vi "Test gRPC cRIO XNET Read DBC Signals.vi"(11 "Test Case In":refnum<class "Test Communicator gRPC.lvclass">) -> (0 "error out":errorcluster, 3 "Test Case Out":refnum<class "Test Communicator gRPC.lvclass">)   [LabVIEW 2025, in "Test Communicator gRPC.lvclass"]
uses:
  Test Communicator gRPC.lvclass
  Test Communicator gRPC.lvclass/Test Communicator gRPC.ctl
  Source/Configure Strategies/gRPC XNET Read Raw CAN Frame Strategy/gRPC XNET Read Raw CAN Frame Strategy.lvclass
  D:/git/HAL/Source/Interfaces/IConfigure/IConfigure.lvclass
  D:/git/HAL/Source/Interfaces/IClose/IClose.lvclass
  D:/git/HAL/Source/Interfaces/IInitialize/IInitialize.lvclass
  D:/git/HAL/HAL-Devices/Source/Configure Strategies/gRPC XNET Read Raw CAN Frame Strategy/gRPC XNET Read Raw CAN Frame Strategy.lvclass
  D:/git/HAL/Source/Interfaces/ICommunicate/ICommunicate.lvclass
  D:/git/HAL/Source/Interfaces/IRunnable/IRunnable.lvclass
  C:/Program Files/National Instruments/LabVIEW 2025/vi.lib/Astemes/LUnit/Test Case.lvclass
  C:/Program Files/National Instruments/LabVIEW 2025/vi.lib/Astemes/LUnit/LUnit Runnable.lvclass
  D:/git/HAL/HAL-Devices/Tests/New folder/Test Communicator gRPC.lvclass
  <vilib>/Astemes/LUnit/Test Case.lvclass
  Source/DBC Communicator/DBC Communicator.lvclass
panel:
  out "Time Stamp":timestamp format="%<%x %.3X>T"
  out "Temp":dbl
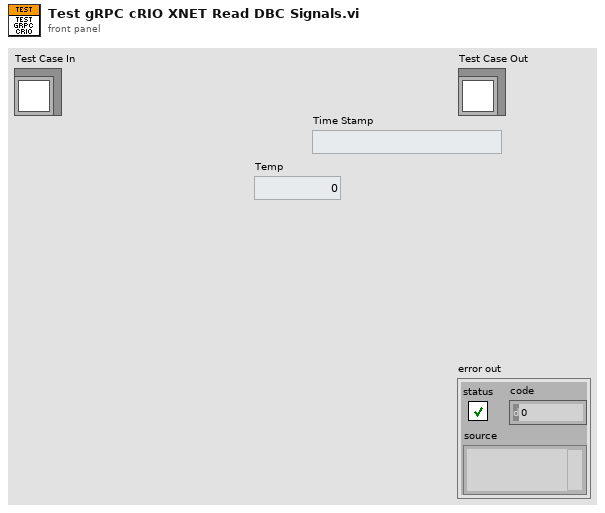
[diagram p1: front panel]
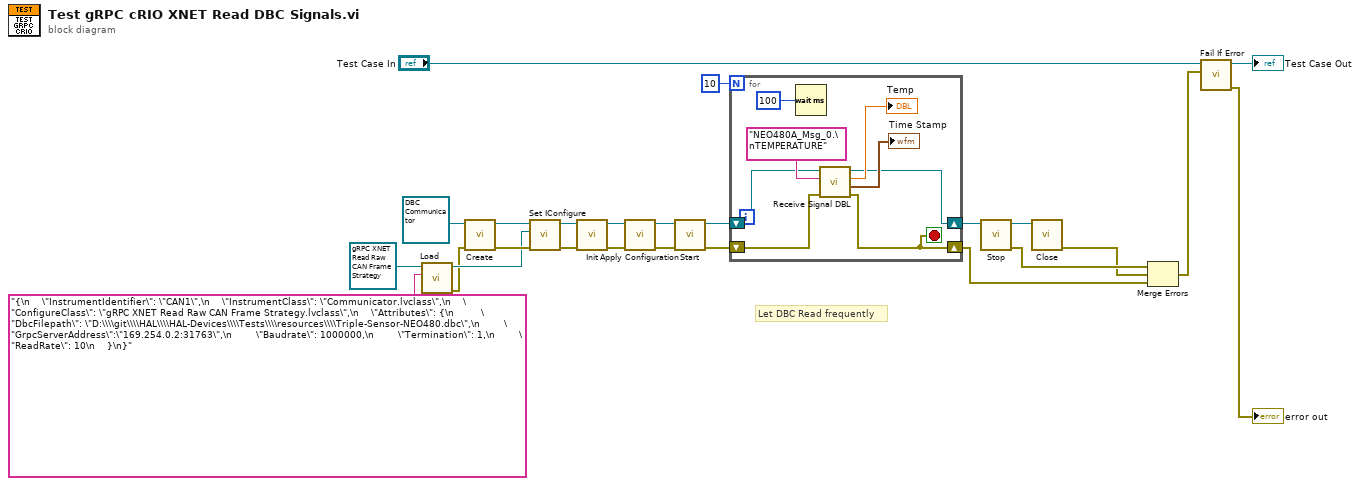
[diagram p0: block diagram]
diagram:
  # "Let DBC Read frequently"
  n1 = call-dynamic "Load.vi"("Source"="{\n    \"InstrumentIdentifier\": \"CAN1\",\n    \"InstrumentClass\": \"Communicator.lvclass\",\n    \"ConfigureClass\": \"gRPC XNET Read Raw CAN Frame Strategy.lvclass\",\n    \"Attributes\": {\n         \"DbcFilepath\": \"D:\\\\git\\\\HAL\\\\HAL-Devices\\\\Tests\\\\resources\\\\Triple-Sensor-NEO480.dbc\",\n        \"GrpcServerAddress\":\"169.254.0.2:31763\",\n        \"Baudrate\": 1000000,\n        \"Termination\": 1,\n        \"ReadRate\": 10\n    }\n}", "gRPC XNET Read Raw CAN Frame Strategy in"=refnum<class "gRPC XNET Read Raw CAN Frame Strategy.lvclass"> refnum ("IConfigure")) -> ("error out"=w8:errorcluster, "gRPC XNET Read Raw CAN Frame Strategy out"=w21:refnum<class "gRPC XNET Read Raw CAN Frame Strategy.lvclass">)  [unwired: 8 in]
  n2 = call-dynamic "Create.vi"("Error In"=w8, "reference in"=refnum<class "DBC Communicator.lvclass"> refnum ("Communicator in")) -> ("Error Out"=w22:errorcluster, "reference out"=w14:refnum<class "DBC Communicator.lvclass">)  [unwired: 8 in]
  n3 = call-dynamic "Set IConfigure.vi"("Error In"=w22, "IConfigure"=w21, "Communicator in"=w14) -> ("Error Out"=w19:errorcluster, "Communicator out"=w1:refnum<class "DBC Communicator.lvclass">)  [unwired: 7 in]
  n4 = call-dynamic "Init.vi"("Error In"=w19, "Communicator in"=w1) -> ("Error Out"=w18:errorcluster, "Communicator out"=w17:refnum<class "DBC Communicator.lvclass">)  [unwired: 8 in]
  n5 = call-dynamic "Apply Configuration.vi"("Error In"=w18, "reference in"=w17) -> ("Error Out"=w12:errorcluster, "reference out"=w7:refnum<class "DBC Communicator.lvclass">)  [unwired: 8 in]
  n6 = call-dynamic "Start.vi"("Error In"=w12, "Communicator in"=w7) -> ("Error Out"=w6:errorcluster, "Communicator out"=w5:refnum<class "DBC Communicator.lvclass">)  [unwired: 8 in]
  n7 = for {
    N: 10 -> [_]
    shift-right: [w26] -> w15
    shift-left: w5 -> [w27]
    shift-right: [w28] -> w4
    shift-left: w6 -> [w30]
    stop <- w28 stop-if-true
    n8 = Wait (ms)(milliseconds to wait=u32 100) -> ()  [unwired: 1 out]
    n9 = call "Receive Signal DBL.vi"("error in"=w30, "Signal Name"="NEO480A_Msg_0.\nTEMPERATURE", "DBC Communication in"=w27) -> ("error out"=w28:errorcluster, "Time Stamp"=→"Time Stamp":timestamp, "Value"=→"Temp":dbl, "DBC Communication out"=w26:refnum<class "DBC Communicator.lvclass">)  [unwired: 5 in]
  }
  n10 = call-dynamic "Stop.vi"("Communicator in"=w15) -> ("Error Out"=w10:errorcluster, "Communicator out"=w13:refnum<class "DBC Communicator.lvclass">)  [unwired: 9 in]
  n11 = call-dynamic "Close.vi"("reference in"=w13) -> ("Error Out"=w2:errorcluster)  [unwired: 9 in, 1 out]
  n12 = Merge Errors(w10, w2, w4) -> (w11:errorcluster)
  n13 = call <vilib>:"Fail If Error.vi"("Assert error"=w11, "LUnit Test Case In"="Test Case In") -> ("error out"=→"error out":errorcluster, "LUnit Test Case Out"=→"Test Case Out":refnum<class "Test Communicator gRPC.lvclass">)  [unwired: 8 in]
